vi "fgv_camera.vi"(7 "cmd":enum16{"ini", "grab", "close"}(ring), 8 "error in":errorcluster, 11 "Image In":T1) -> (0 "error out":errorcluster, 3 "Image Out":T1)   [LabVIEW 2019]
uses:
  <vilib>/vision/Image Controls.llb/IMAQ Image.ctl
  <vilib>/vision/driver/NI_Vision_Acquisition_Software.lvlib
  <resource>/objmgr/imaqdx.rc
panel:
  in  "camera file":path
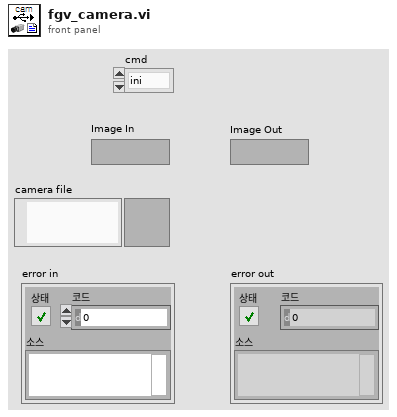
[diagram p1: front panel]
types:
  T1 = typedef "IMAQ Image.ctl" = refnum<image>
  T2 = typedef "IMAQdx.ctl" = refnum<k21>
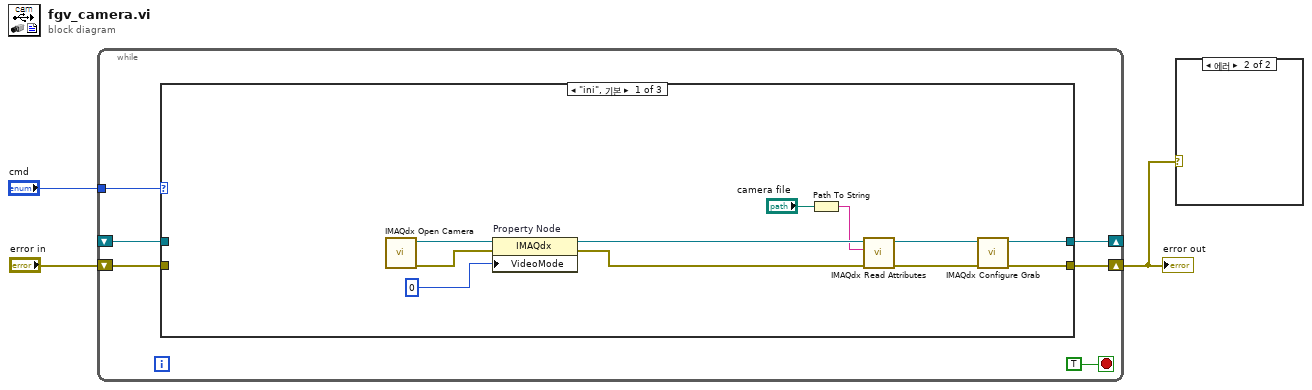
[diagram p0: block diagram]
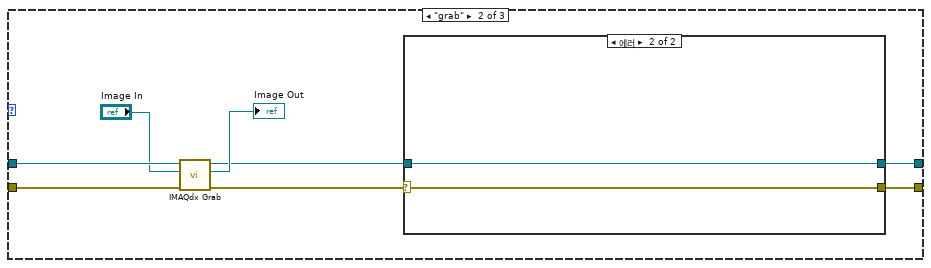
[diagram p3: hidden frame]
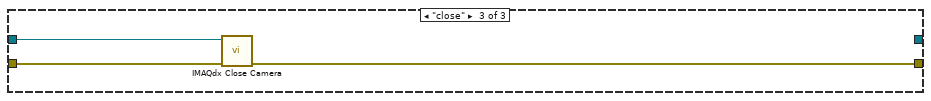
[diagram p5: hidden frame]
diagram:
  n1 = while {
    tunnel: "cmd" -> [w8]
    shift-right: [w6] -> w1
    shift-left: "error in" -> [w7]
    shift-right: [w5] -> _
    shift-left: _ -> [w4]
    stop <- TRUE stop-if-true
    n2 = case shown="\"ini\", 기본" w8 {
      tunnel: w7 -> [_ w27 w34]
      tunnel: [w19 w23 w33] -> w6
      tunnel: [w20 w22 _] -> w5
      tunnel: w4 -> [_ w28 w35]
      frame "ini", Default {
        n3 = call <vilib>:"IMAQdx Open Camera.vi"() -> ("error out"=w17:errorcluster, "Session Out"=w18:T2)  [unwired: 10 in]
        n4 = property on="Property Node" class="IMAQdx"(reference=w18, error in=w17, "VideoMode"=u32 0) -> (reference out=w14:T2, error out=w13:errorcluster)
        n5 = Path To String(path="camera file") -> (string=w12:string)
        n6 = call <vilib>:"IMAQdx Read Attributes.vi"("error in"=w13, "Filename"=w12, "Session In"=w14) -> ("error out"=w15:errorcluster, "Session Out"=w16:T2)  [unwired: 7 in]
        n7 = call <vilib>:"IMAQdx Configure Grab.vi"("error in"=w15, "Session In"=w16) -> ("error out"=w19:errorcluster, "Session Out"=w20:T2)  [unwired: 8 in]
      }
      frame "grab" {
        n8 = call <vilib>:"IMAQdx Grab.vi"("error in"=w27, "Image In"="Image In", "Session In"=w28) -> ("error out"=w24:errorcluster, "Image Out"=→"Image Out":T1, "Session Out"=w21:T2)  [unwired: 5 in, 1 out]
        n9 = case shown="에러" w24 {
          selector: w24 -> [w30 w32]
          tunnel: [w30 w32] -> w23
          tunnel: [w29 w31] -> w22
          tunnel: w21 -> [w29 w31]
          frame No Error {
          }
          frame Error {
          }
        }
      }
      frame "close" {
        n10 = call <vilib>:"IMAQdx Close Camera.vi"("error in"=w34, "Session In"=w35) -> ("error out"=w33:errorcluster)  [unwired: 9 in]
      }
    }
  }
  "error out" <- w1
  n11 = case shown="에러" w1 {
    frame No Error {
    }
    frame Error {
    }
  }
